vi "waveform player control.vi"(0 "type":T1(ring), 1 "notifier name":string="wave out", 2 "waveform":u8[](array[slide]) scale=0.0..255.0, 3 "volume":i16(slide) scale=0.0..32767.0) -> ()   [LabVIEW 2009]
uses:
  event notifier.ctl
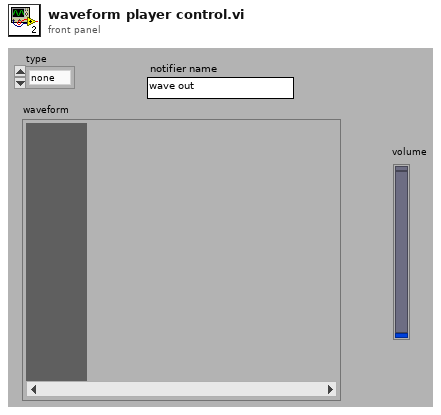
[diagram p1: front panel]
types:
  T1 = enum8{"none", "end", "start", "pause", "update", "volume"}
  T2 = typedef "event notifier.ctl" = cluster{"type":enum8{"none", "end", "start", "pause", "update", "volume"}, "message":string}
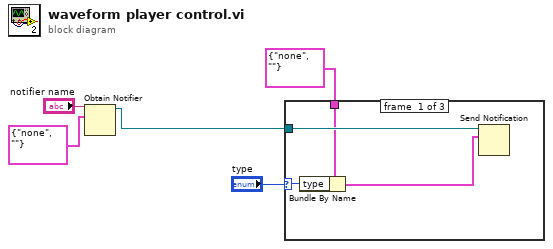
[diagram p0: block diagram]
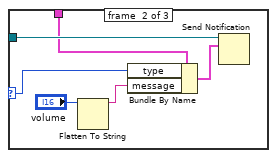
[diagram p2: hidden frame]
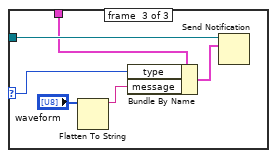
[diagram p3: hidden frame]
diagram:
  n1 = Obtain Notifier(name (unnamed)="notifier name", notification data type=T2 {"type"=enum."none", "message"=""} ("notification")) -> (notifier out=w4:refnum<notifier>)  [unwired: 2 in, 2 out]
  n2 = case shown="\"volume\"" "type" {
    selector: "type" -> [w6 w10 w16]
    tunnel: T2 {"type"=enum."none", "message"=""} ("notification") -> [w8 w14 w20]
    tunnel: w4 -> [w9 w15 w21]
    frame #0 {
      n3 = Bundle By Name(cluster=w8, "type"=w6) -> (w7:T2)
      n4 = Send Notification(notification=w7, notifier=w9) -> ()  [unwired: 1 in, 2 out]
    }
    frame #1 {
      n5 = Flatten To String(anything="volume") -> (data string=w11:string)  [unwired: 3 in, 2 out]
      n6 = Bundle By Name(cluster=w14, "type"=w10, "message"=w11) -> (w13:T2)
      n7 = Send Notification(notification=w13, notifier=w15) -> ()  [unwired: 1 in, 2 out]
    }
    frame #2 {
      n8 = Flatten To String(anything="waveform") -> (data string=w18:string)  [unwired: 3 in, 2 out]
      n9 = Bundle By Name(cluster=w20, "type"=w16, "message"=w18) -> (w19:T2)
      n10 = Send Notification(notification=w19, notifier=w21) -> ()  [unwired: 1 in, 2 out]
    }
  }
